vi "InterpolateStage1.vi"(8 "valid in":bool, 11 "Data in":fxp<+/-,16,14>[](array[numeric])=[0.0, 0.0]) -> (0 "valid out":bool, 3 "Data out":fxp<+/-,16,14>[](array[numeric]))   [LabVIEW 2013]
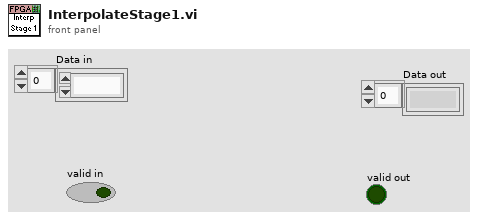
[diagram p1: front panel]
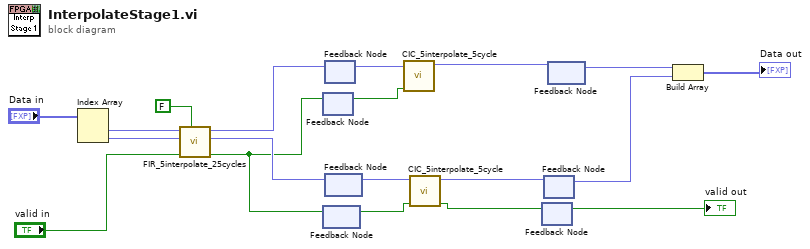
[diagram p0: block diagram]
diagram:
  n1 = Index Array(array="Data in") -> (element #1=w18:fxp<+/-,16,14>, element #2=w17:fxp<+/-,16,14>)  [unwired: 2 in]
  n2 = call "FIR_5interpolate_25cycles.vi"("reset"=FALSE, "valid in"="valid in", "Q in"=w17, "I in"=w18) -> ("valid out"=w12:bool, "Q out"=w13:fxp<+/-,16,14>, "I out"=w14:fxp<+/-,16,14>)  [unwired: 4 in, 1 out]
  n3 = feedback #1() -> (w10:bool)  [unwired: 1 in]
  n4 = feedback-in #1(w12) -> ()
  n5 = feedback #2() -> (w6:bool)  [unwired: 1 in]
  n6 = feedback-in #2(w12) -> ()
  n7 = feedback-in #3(w14) -> ()
  n8 = feedback #3() -> (w11:fxp<+/-,16,14>)  [unwired: 1 in]
  n9 = feedback #4() -> (w7:fxp<+/-,16,14>)  [unwired: 1 in]
  n10 = feedback-in #4(w13) -> ()
  n11 = call "CIC_5interpolate_5cycle.vi"("valid in"=w10, "Data in"=w11) -> ("Data out"=w9:fxp<+/-,16,14>)  [unwired: 8 in, 1 out]
  n12 = call "CIC_5interpolate_5cycle.vi"("valid in"=w6, "Data in"=w7) -> ("valid out"=w4:bool, "Data out"=w5:fxp<+/-,16,14>)  [unwired: 8 in]
  n13 = feedback #5() -> (→"valid out":bool)  [unwired: 1 in]
  n14 = feedback-in #5(w4) -> ()
  n15 = feedback #6() -> (w2:fxp<+/-,16,14>)  [unwired: 1 in]
  n16 = feedback-in #6(w5) -> ()
  n17 = feedback #7() -> (w8:fxp<+/-,16,14>)  [unwired: 1 in]
  n18 = feedback-in #7(w9) -> ()
  n19 = Build Array(w8, w2) -> (→"Data out":fxp<+/-,16,14>[])
